vi "Excel_Print.vi"(0 "Excel._Worksheet":refnum<k7>, 7 "printer name (default)":string, 9 "number of copies (1)":i32, 11 "error in (no error)":errorcluster) -> (15 "error out":errorcluster)   [LabVIEW 2010, in "NI_ReportGenerationToolkit.lvlib"]
uses:
  <vilib>/addons/_office/NI_ReportGenerationToolkit.lvlib
  <vilib>/Utility/NIReport.llb/NI_ReportGenerationCore.lvlib
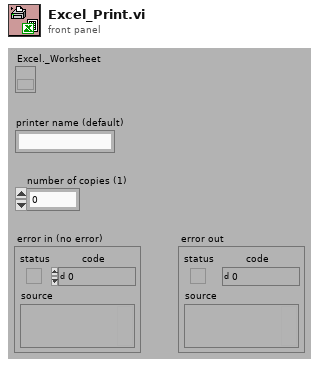
[diagram p1: front panel]
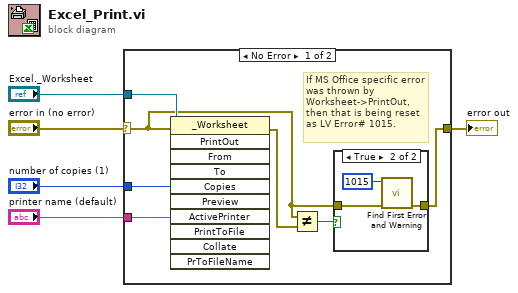
[diagram p0: block diagram]
diagram:
  n1 = case shown="No Error" "error in (no error)" {
    selector: "error in (no error)" -> [w6 w17]
    tunnel: [w12 w17] -> w5
    tunnel: "Excel._Worksheet" -> [w11 _]
    tunnel: "printer name (default)" -> [w10 _]
    tunnel: "number of copies (1)" -> [w9 _]
    frame No Error {
      # "If MS Office specific error was thrown by Worksheet->PrintOut, then that is being reset as LV Error# 1015."
      n2 = invoke class="_Worksheet" method="PrintOut"(reference=w11, error in=w6, "Copies"=w9, "ActivePrinter"=w10) -> (error out=w8:errorcluster)  [unwired: 7 in, 10 out]
      n3 = Not Equal?(x=w6, y=w8) -> (x != y?=w7:bool)
      n4 = case shown="True" w7 {
        tunnel: w6 -> [w13 w15]
        tunnel: [w13 w14] -> w12
        frame False {
        }
        frame True {
          n5 = call <vilib>:"Find First Error and Warning.vi"("error in (no error)"=w15, "error code"=1015) -> ("error out"=w14:errorcluster)  [unwired: 4 in, 1 out]
        }
      }
    }
    frame Error {
    }
  }
  "error out" <- w5
